vi "In_S6F2.vi"(8 "error in (no error)":errorcluster, 11 "S6 Message Class in":refnum<class "S6 Message Class.lvclass">) -> (0 "error out":errorcluster, 1 "OK?":bool, 2 "ACK":bool, 3 "S6 Message Class out":refnum<class "S6 Message Class.lvclass">)   [LabVIEW 2020, in "SECS Communication.lvlib" / "S6 Message Class.lvclass"]
uses:
  S6 Message Class.lvclass
  D:/Dropbox/SECS/SECS_GEM v1.0.6/Com/SECS Communication/SECS-II Class/SECS-II Class.lvclass
  SECS-II Class/SECS-II Class.lvclass/SECS-II Class.ctl
  SECS-II Class/Variant To Data_Binary.vi
  SECS-II Class/SECS-II Class.lvclass
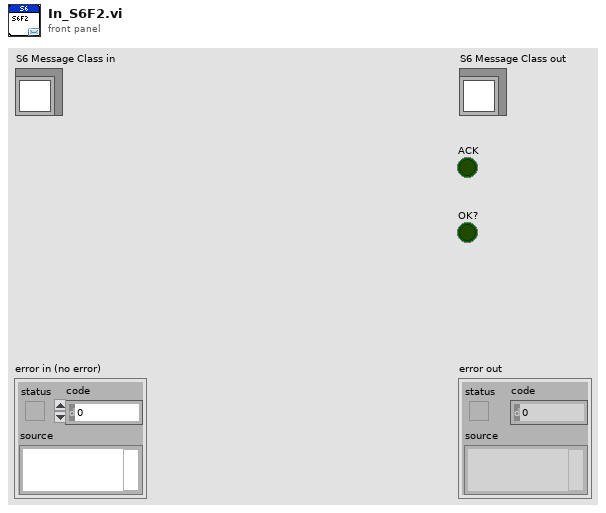
[diagram p1: front panel]
types:
  T1 = typedef "SECS Communication.lvlib/SECS-II Class.lvclass/Message Data.ctl" = cluster{"Index":i32, "Data Item Format":T2, "Format Code":T3, "Parent Index":i32, "Child Index":i32[], "Data":variant}
  T2 = typedef "SECS Communication.lvlib/SECS-II Class.lvclass/Data Item Format.ctl" = enum16{"Data Type", "Value"}
  T3 = typedef "SECS Communication.lvlib/SECS-II Class.lvclass/Format Code.ctl" = enum16{"L", "A", "B", "Boolean", "J", "I1", "I2", "I4", "I8", "U1", "U2", "U4", "U8", "F4", "F8", "Char"}
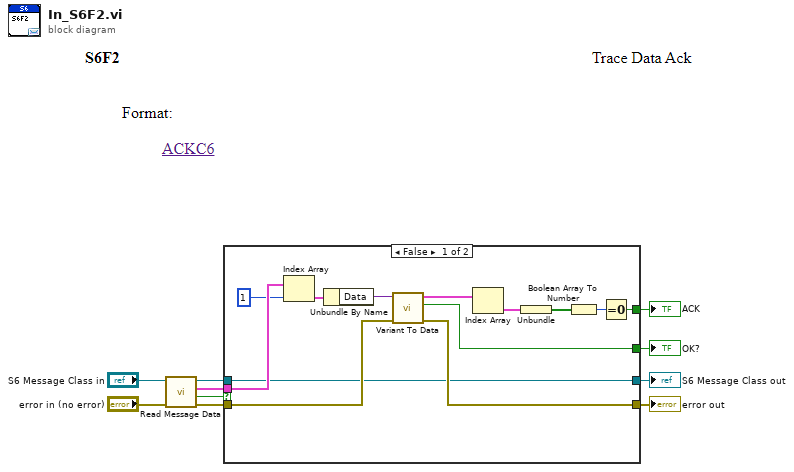
[diagram p0: block diagram]
diagram:
  n1 = call "Read Message Data.vi"("error in (no error)"="error in (no error)", "SECS-II Class in"="S6 Message Class in") -> ("error out"=w7:errorcluster, "Empty?"=w3:bool, "Message Data"=w8:T1[], "SECS-II Class out"=w4:refnum<class "S6 Message Class.lvclass">)  [unwired: 6 in]
  n2 = case shown="False" w3 {
    tunnel: w8 -> [w23 _]
    tunnel: w7 -> [w19 w25]
    tunnel: [w18 w25] -> w6
    tunnel: [w13 _] -> w5
    tunnel: w4 -> [w12 w24]
    tunnel: [w12 w24] -> w2
    tunnel: [w11 _] -> w1
    frame False {
      n3 = Index Array(array=w23, index=1) -> (element=w21:T1)
      n4 = Unbundle By Name(w21) -> ("Data"=w20:variant)
      n5 = call-poly "Variant To Data.vi"("error in (no error)"=w19, "Variant"=w20) -> ("error out"=w18:errorcluster, "OK?"=w11:bool, "Data Cluster"=w17:cluster{"Data":bool[]}[])  [unwired: 7 in]
      n6 = Index Array(array=w17) -> (element=w16:cluster{"Data":bool[]})  [unwired: 1 in]
      n7 = Unbundle(w16) -> ("Data"=w15:bool[])
      n8 = Boolean Array To Number(Boolean array=w15) -> (number=w14:u32)
      n9 = Equal To 0?(x=w14) -> (x = 0?=w13:bool)
    }
    frame True {
    }
  }
  "error out" <- w6
  "S6 Message Class out" <- w2
  "ACK" <- w5
  "OK?" <- w1
